vi "Write T Controller Settings.vi"(4 "New PID":cluster{"P":dbl, "I":dbl, "D":dbl}, 6 "Heater level":dbl, 7 "Set point":dbl, 8 "error in (no error)":errorcluster, 9 "New Heater mode":T1(ring), 10 "Heater range":dbl, 11 "Neocera LTC-21 in":refnum<class "Neocera LTC-21.lvclass">) -> (0 "error out":errorcluster, 3 "Neocera LTC-21 out":refnum<class "Neocera LTC-21.lvclass">)   [LabVIEW 2015, in "Neocera LTC-21.lvclass"]
uses:
  Neocera LTC-21.lvclass
  Instrument/Instrument.lvclass
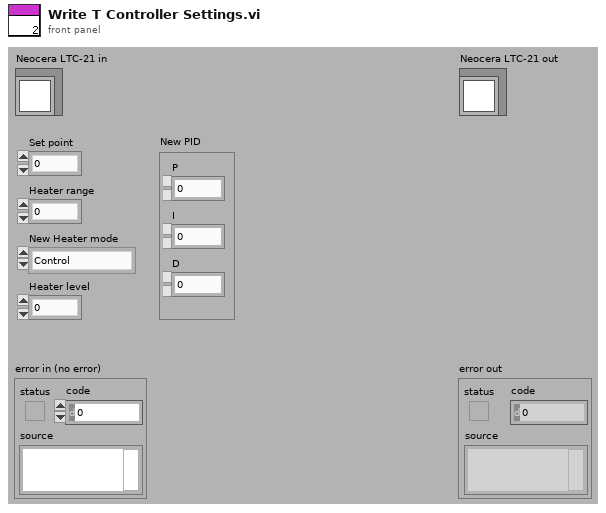
[diagram p1: front panel]
types:
  T1 = enum16{"Control", "Monitor", "Manual Heat", "Controller is in OFF mode", "Autotune is in progress"}
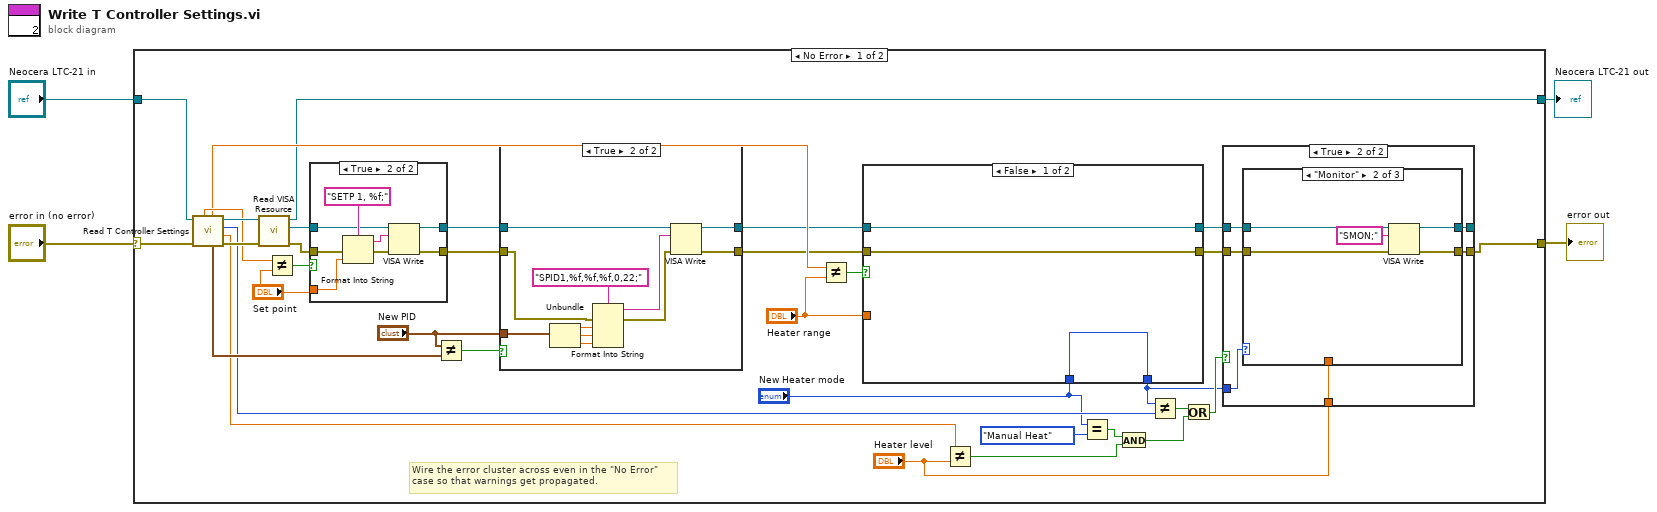
[diagram p0: block diagram]
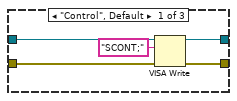
[diagram p4: hidden frame]
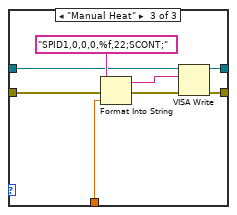
[diagram p5: hidden frame]
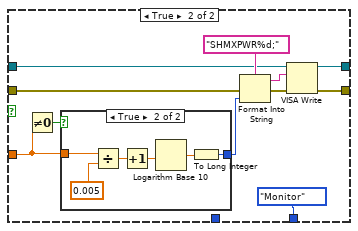
[diagram p6: hidden frame]
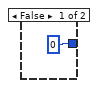
[diagram p7: hidden frame]
diagram:
  n1 = case shown="No Error" "error in (no error)" {
    selector: "error in (no error)" -> [w28 w110]
    tunnel: [w22 w110] -> w3
    tunnel: [w26 w109] -> w1
    tunnel: "Neocera LTC-21 in" -> [w27 w109]
    frame No Error {
      # "Wire the error cluster across even in the \"No Error\"\ncase so that warnings get propagated."
      n2 = call-dynamic "Read T Controller Settings.vi"("error in (no error)"=w28, "Neocera LTC-21 in"=w27) -> ("error out"=w37:errorcluster, "Heater level"=w14:dbl, "Heater mode"=w11:T1, "Neocera LTC-21 out"=w38:refnum<class "Neocera LTC-21.lvclass">, "PID"=w21:cluster{"P":dbl, "I":dbl, "D":dbl}, "Hater range"=w30:dbl, "Set point"=w36:dbl)  [unwired: 3 in]
      n3 = call "Read VISA Resource.vi"("error in (no error)"=w37, "Instrument.lvclass in"=w38) -> ("error out"=w34:errorcluster, "VISA Resource"=w32:refnum<visa-resource-name>, "Instrument.lvclass out"=w26:refnum<class "Neocera LTC-21.lvclass">)  [unwired: 7 out]
      n4 = Not Equal?(x=w36, y="Set point") -> (x != y?=w35:bool)
      n5 = case shown="True" w35 {
        tunnel: w34 -> [w100 w106]
        tunnel: "Set point" -> [_ w107]
        tunnel: w32 -> [w99 w104]
        tunnel: [w100 w103] -> w19
        tunnel: [w99 w102] -> w17
        frame False {
        }
        frame True {
          n6 = Format Into String(format string="SETP 1, %f;" ("write buffer"), error in=w106, w107) -> (resulting string=w101:string, error out=w105:errorcluster)  [unwired: 1 in]
          n7 = VISA Write(VISA resource name=w104, write buffer=w101, error in (no error)=w105) -> (VISA resource name out=w102:refnum<visa-resource-name>, error out=w103:errorcluster)  [unwired: 1 out]
        }
      }
      n8 = Not Equal?(x="New PID", y=w21) -> (x != y?=w20:bool)
      n9 = case shown="True" w20 {
        tunnel: w19 -> [w40 w46]
        tunnel: [w40 w44] -> w18
        tunnel: w17 -> [w39 w41]
        tunnel: [w39 w43] -> w16
        tunnel: "New PID" -> [_ w51]
        frame False {
        }
        frame True {
          n10 = Unbundle(w51) -> ("P"=w50:dbl, "I"=w49:dbl, "D"=w48:dbl)
          n11 = Format Into String(format string="SPID1,%f,%f,%f,0,22;", error in=w46, w50, w49, w48) -> (resulting string=w42:string, error out=w45:errorcluster)  [unwired: 1 in]
          n12 = VISA Write(VISA resource name=w41, write buffer=w42, error in (no error)=w45) -> (VISA resource name out=w43:refnum<visa-resource-name>, error out=w44:errorcluster)  [unwired: 1 out]
        }
      }
      n13 = Not Equal?(x=w30, y="Heater range") -> (x != y?=w31:bool)
      n14 = case shown="False" w31 {
        tunnel: w18 -> [w80 w90]
        tunnel: "Heater range" -> [_ w84]
        tunnel: w16 -> [w79 w88]
        tunnel: [w80 w87] -> w23
        tunnel: [w79 w86] -> w24
        tunnel: [w78 T1."Monitor" ("New Heater mode")] -> w6
        tunnel: "New Heater mode" -> [w78 _]
        frame False {
        }
        frame True {
          n15 = Not Equal To 0?(x=w84) -> (x != 0?=w85:bool)
          n16 = case shown="True" w85 {
            tunnel: w84 -> [_ w97]
            tunnel: [0 w94] -> w83
            frame False {
            }
            frame True {
              n17 = Divide(x=w97, y=0.005) -> (x/y=w96:dbl)
              n18 = Increment(x=w96) -> (x+1=w93:dbl)
              n19 = Logarithm Base 10(1:w93) -> (0:w95:dbl)
              n20 = To Long Integer(number=w95) -> (32bit integer=w94:i32)
            }
          }
          n21 = Format Into String(format string="SHMXPWR%d;" ("write buffer"), error in=w90, w83) -> (resulting string=w82:string, error out=w89:errorcluster)  [unwired: 1 in]
          n22 = VISA Write(VISA resource name=w88, write buffer=w82, error in (no error)=w89) -> (VISA resource name out=w86:refnum<visa-resource-name>, error out=w87:errorcluster)  [unwired: 1 out]
        }
      }
      n23 = Not Equal?(x=w14, y="Heater level") -> (x != y?=w9:bool)
      n24 = Equal?(x="New Heater mode", y=T1."Manual Heat" ("New Heater mode")) -> (x = y?=w10:bool)
      n25 = And(x=w10, y=w9) -> (x .and. y?=w7:bool)
      n26 = Not Equal?(x=w6, y=w11) -> (x != y?=w29:bool)
      n27 = Or(x=w29, y=w7) -> (x .or. y?=w8:bool)
      n28 = case shown="True" w8 {
        tunnel: w6 -> [_ w59]
        tunnel: w23 -> [w53 w58]
        tunnel: w24 -> [w52 w57]
        tunnel: [w52 w56] -> _
        tunnel: [w53 w55] -> w22
        tunnel: "Heater level" -> [_ w54]
        frame False {
        }
        frame True {
          n29 = case shown="\"Monitor\"" w59 {
            tunnel: w58 -> [w64 w69 w75]
            tunnel: w57 -> [w63 w68 w71]
            tunnel: [w61 w66 w74] -> w55
            tunnel: [w60 w65 w70] -> w56
            tunnel: w54 -> [_ _ w72]
            frame "Control", Default {
              n30 = VISA Write(VISA resource name=w63, write buffer="SCONT;", error in (no error)=w64) -> (VISA resource name out=w60:refnum<visa-resource-name>, error out=w61:errorcluster)  [unwired: 1 out]
            }
            frame "Monitor" {
              n31 = VISA Write(VISA resource name=w68, write buffer="SMON;", error in (no error)=w69) -> (VISA resource name out=w65:refnum<visa-resource-name>, error out=w66:errorcluster)  [unwired: 1 out]
            }
            frame "Manual Heat" {
              n32 = Format Into String(format string="SPID1,0,0,0,%f,22;SCONT;", error in=w75, w72) -> (resulting string=w76:string, error out=w77:errorcluster)  [unwired: 1 in]
              n33 = VISA Write(VISA resource name=w71, write buffer=w76, error in (no error)=w77) -> (VISA resource name out=w70:refnum<visa-resource-name>, error out=w74:errorcluster)  [unwired: 1 out]
            }
          }
        }
      }
    }
    frame Error {
    }
  }
  "error out" <- w3
  "Neocera LTC-21 out" <- w1
